vi "basic_movement.vi"() -> ()   [LabVIEW 2019]
uses:
  <vilib>/myRIO/Common/Instrument Driver Framework/myRIO v1.0/Encoder/typedefs/Encoder Signal Mode.ctl
  <vilib>/myRIO/Instrument Drivers/Onboard IO/AI/typedefs/AI Reference.ctl
  <vilib>/myRIO/Common/Instrument Driver Framework/Utilities/typedefs/myRIO Generic Hardware Reference.ctl
  <vilib>/myRIO/Common/Instrument Driver Framework/Utilities/typedefs/Hardware Version Enum.ctl
  <vilib>/myRIO/Common/Instrument Driver Framework/Utilities/typedefs/myRIO v1.0 Reference.ctl
  <vilib>/myRIO/Common/Instrument Driver Framework/Utilities/typedefs/Generic FPGA Reference.ctl
  <vilib>/myRIO/Common/Instrument Driver Framework/myRIO v1.0/AI/typedefs/AI Channels List.ctl
  <vilib>/myRIO/Common/Instrument Driver Framework/myRIO v1.0/AI/typedefs/AI Channels Enum.ctl
  <vilib>/myRIO/Common/Instrument Driver Framework/Utilities/typedefs/Analog Scaling Constants List.ctl
  <vilib>/myRIO/Common/Instrument Driver Framework/Utilities/typedefs/Analog Scaling Constants.ctl
  <vilib>/userDefined/High Color/nirio_resource_hc.ctl
  <vilib>/myRIO/Instrument Drivers/Onboard IO/AO/typedefs/AO Reference.ctl
  <vilib>/myRIO/Common/Instrument Driver Framework/myRIO v1.0/AO/typedefs/AO Channels List.ctl
  <vilib>/myRIO/Common/Instrument Driver Framework/myRIO v1.0/AO/typedefs/AO Channels Enum.ctl
  Shared VIs/TypeDef_TDMS_States.ctl
  <vilib>/Platform/TimedLoop/XDataNode/timing_clust.ctl
  <vilib>/Platform/TimedLoop/XDataNode/nitl_modes.ctl
  <vilib>/Platform/TimedLoop/XDataNode/wakeup.ctl
  <vilib>/myRIO/Common/Instrument Driver Framework/myRIO v1.0/AI/vis/myRIO v1.1 Open AI.vi
  <vilib>/myRIO/Common/Instrument Driver Framework/myRIO v1.0/AO/vis/myRIO v1.1 Open AO.vi
  <vilib>/myRIO/Common/Instrument Driver Framework/Utilities/vis/Validate Channels.vi
  <vilib>/myRIO/Common/Instrument Driver Framework/myRIO v1.0/AI/vis/myRIO v1.0 Reserve AI.vi
  <vilib>/myRIO/Common/Instrument Driver Framework/myRIO v1.0/AO/vis/myRIO v1.0 Reserve AO.vi
  <vilib>/myRIO/Common/Instrument Driver Framework/myRIO v1.0/AI/vis/myRIO v1.0 Close AI.vi
  <vilib>/myRIO/Common/Instrument Driver Framework/myRIO v1.0/Encoder/vis/myRIO v1.0 Close Encoder.vi
  <vilib>/myRIO/Common/Instrument Driver Framework/myRIO v1.0/AO/vis/myRIO v1.0 Close AO.vi
  <vilib>/myRIO/Common/Instrument Driver Framework/myRIO v1.0/AI/vis/myRIO v1.0 Build MUX Configuration AI.vi
  <vilib>/myRIO/Common/Instrument Driver Framework/myRIO v1.0/Resource Manager/vis/myRIO v1.0 Reserve Channel List.vi
  <vilib>/myRIO/Common/Instrument Driver Framework/myRIO v1.0/AO/vis/myRIO v1.0 Build MUX Configuration AO.vi
  <vilib>/myRIO/Common/Instrument Driver Framework/myRIO v1.0/AI/vis/myRIO v1.0 Unreserve AI.vi
  <vilib>/myRIO/Common/Instrument Driver Framework/myRIO v1.0/Encoder/vis/myRIO v1.0 Unreserve Encoder.vi
  <vilib>/myRIO/Common/Instrument Driver Framework/myRIO v1.0/AO/vis/myRIO v1.0 Unreserve AO.vi
  <vilib>/myRIO/Common/Instrument Driver Framework/myRIO v1.0/Resource Manager/vis/myRIO v1.0 Reserve Channel.vi
  <vilib>/myRIO/Common/Instrument Driver Framework/myRIO v1.0/Resource Manager/vis/myRIO v1.0 Unreserve Channel.vi
  <vilib>/myRIO/Common/Instrument Driver Framework/myRIO v1.0/Resource Manager/vis/myRIO v1.0 Unreserve Channel List.vi
  <vilib>/myRIO/Common/Instrument Driver Framework/myRIO v1.0/Encoder/vis/myRIO v1.0 Build MUX Configuration Encoder.vi
  <vilib>/myRIO/Common/Instrument Driver Framework/myRIO v1.0/Resource Manager/vis/myRIO v1.0 Build Mutex Name.vi
  <vilib>/myRIO/Common/Instrument Driver Framework/myRIO v1.0/Resource Manager/vis/myRIO v1.0 Create Configuration List.vi
  <vilib>/Utility/VariantDataType/GetNumericInfo.vi
  <vilib>/Utility/error.llb/Error Cluster From Error Code.vi
  <vilib>/myRIO/Common/Instrument Driver Framework/myRIO v1.0/myRIO v1.1 Open.vi
  <vilib>/myRIO/Common/Instrument Driver Framework/myRIO v1.0/AO/vis/myRIO v1.0 Get Scaling Constants AO.vi
  <vilib>/myRIO/Common/Instrument Driver Framework/Utilities/vis/IO Manager.vi
  <vilib>/myRIO/Common/Instrument Driver Framework/Utilities/vis/Configuration Manager.vi
  <vilib>/myRIO/Common/Instrument Driver Framework/myRIO v1.0/myRIO v1.0 Close.vi
  <vilib>/myRIO/Common/Instrument Driver Framework/myRIO v1.0/AO/vis/myRIO v1.0 Write AO.vi
  <vilib>/myRIO/Common/Instrument Driver Framework/myRIO v1.0/AI/vis/myRIO v1.0 Get Scaling Constants AI.vi
  <vilib>/myRIO/Common/Instrument Driver Framework/myRIO v1.0/AI/vis/myRIO v1.0 Read AI.vi
  <vilib>/myRIO/Common/Instrument Driver Framework/myRIO v1.0/Encoder/vis/myRIO v1.0 Read Encoder.vi
  <vilib>/myRIO/Common/Instrument Driver Framework/myRIO v1.0/Encoder/vis/myRIO v1.0 Enable Encoder.vi
  <vilib>/myRIO/Common/Instrument Driver Framework/myRIO v1.0/Encoder/vis/myRIO v1.0 Shutdown Encoder.vi
  <vilib>/myRIO/Common/Instrument Driver Framework/myRIO v1.0/Resource Manager/vis/myRIO v1.0 Configure IO.vi
  <vilib>/myRIO/Instrument Drivers/Onboard IO/AO/vis/myRIO AO Open.xnode
  <vilib>/myRIO/Instrument Drivers/Onboard IO/AI/vis/myRIO AI Open.xnode
  <vilib>/Platform/TimedLoop/XDataNode/XDataNode.xnode
  <vilib>/myRIO/Instrument Drivers/Onboard IO/Encoder/Encoder.lvlib
  <vilib>/myRIO/Instrument Drivers/Onboard IO/AO/AO.lvlib
  <vilib>/Platform/TimedLoop/XDataNode/XDNodeRunTimeDep.lvlib
  <vilib>/myRIO/Instrument Drivers/Onboard IO/AI/AI.lvlib
panel:
  in  "Save data?":bool
  in  "Stop Saving Data":bool
  in  "Filename Data Save":string
  in  "START":bool
  in  "Motor Input Voltage [V]":dbl
  out "Current (A)":dbl
  out "Loop Number (dt = 1 ms)":dbl
  in  "STOP":bool
  out "Elapsed Time (ms)":dbl
  out "Initial Time (ms)":dbl
  out "Encoder Position (deg)":dbl
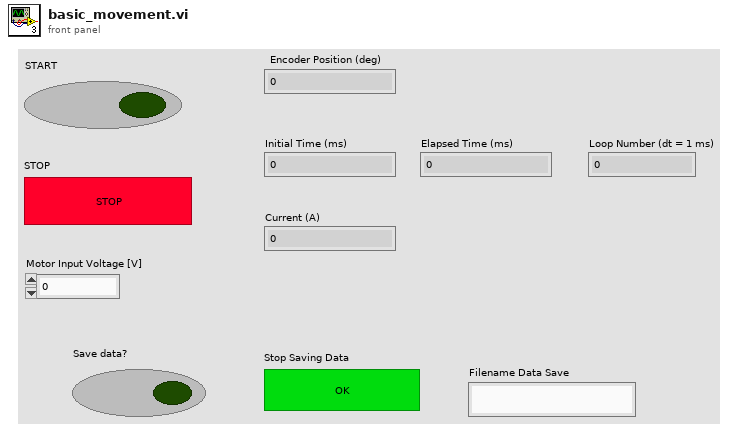
[diagram p1: front panel]
types:
  T1 = typedef "nirio_resource_hc.ctl" = tag
  T2 = typedef "Hardware Version Enum.ctl" = enum16{"Unknown", "myRIO-1900", "myRIO-1950", "roboRIO", "NI ELVIS RIO CM", "ELVIS III"}
  T3 = typedef "TypeDef_TDMS_States.ctl" = enum16{"WaitingForCreate", "Create", "Buffering", "Flushing", "Write", "Close"}
  T4 = enum16{"open", "open or create", "create or replace", "create", "open (read-only)"}
  T5 = typedef "XDNodeRunTimeDep.lvlib/timing_clust.ctl" = cluster{"Expected End [f-1]":u64, "Actual End [f-1]":u64, "Finished Late? [f-1]":bool, "Expected End [i-1]":u64, "Actual End [i-1]":u64, "Finished Late? [i-1]":bool, "Expected Start [i]":u64, "Actual Start [i]":u64, "Expected Start [f]":u64, "Actual Start [f]":u64, "Source Name":string, "Structure Name":string, "Period":i64, "Deadline":i64, "Offset":i64, "Start":i64, "Priority":i32, "Timeout":i32, "Mode":T6, "Wakeup Reason":T7, "Error":errorcluster, "Source Type":string, "Secondary Source Type":string, "Global End Time":u64, "Global Start Time":u64, "Frame Duration":u64, "Iteration Duration":u64, "Assigned CPU":i32, "I/O Scan Engine Mode":u32}
  T6 = typedef "XDNodeRunTimeDep.lvlib/nitl_modes.ctl" = enum32{"No Change", "Process missed periods, maintain original phase", "Discard missed periods, maintain original phase", "Process missed periods, ignore original phase", "Discard missed periods, ignore original phase"}
  T7 = typedef "XDNodeRunTimeDep.lvlib/wakeup.ctl" = enum32{"Normal", "Aborted", "Asynchronous wakeup", "Timing source error", "Timed loop error", "Timeout"}
  T8 = typedef "Encoder Signal Mode.ctl" = enum16{"Quadrature phase signal", "Step and direction signal"}
  T9 = typedef "AO.lvlib/AO Reference.ctl" = cluster{"myRIO Reference":T10, "AO Channel List":T13, "AO Scaling Constant List":T15}
  T10 = typedef "myRIO Generic Hardware Reference.ctl" = cluster{"myRIO Model":T2, "myRIO Hardware Reference":T11}
  T11 = typedef "myRIO v1.0 Reference.ctl" = cluster{"Generic FPGA Reference":T12, "Allow multiple opens":bool}
  T12 = typedef "Generic FPGA Reference.ctl" = refnum<k20>
  T13 = typedef "AO Channels List.ctl" = T14[]
  T14 = typedef "AO Channels Enum.ctl" = enum16{"Not Connected", "AudioOut/Left", "AudioOut/Right", "C/AO0", "C/AO1", "A/AO0", "A/AO1", "B/AO0", "B/AO1"}
  T15 = typedef "Analog Scaling Constants List.ctl" = T16[]
  T16 = typedef "Analog Scaling Constants.ctl" = cluster{"LSB Weight (Volts)":dbl, "Offset (Volts)":dbl, "Signed?":bool}
  T17 = typedef "AI.lvlib/AI Reference.ctl" = cluster{"myRIO Reference":T10, "AI Channels List":T18, "AI Scaling Constants List":T15}
  T18 = typedef "AI Channels List.ctl" = T19[]
  T19 = typedef "AI Channels Enum.ctl" = enum16{"Not Connected", "AudioIn/Left", "AudioIn/Right", "C/AI0", "C/AI1", "A/AI0", "A/AI1", "A/AI2", "A/AI3", "A/AI4", "A/AI5", "A/AI6", "A/AI7", "B/AI0", "B/AI1", "B/AI2", "B/AI3", "B/AI4", "B/AI5", "B/AI6", "B/AI7", "AI/AI0", "AI/AI1", "AI/AI2", "AI/AI3", "A/AI0 (DIFF)", "A/AI1 (DIFF)", "A/AI2 (DIFF)", "A/AI3 (DIFF)", "B/AI0 (DIFF)", "B/AI1 (DIFF)", "B/AI2 (DIFF)", "B/AI3 (DIFF)"}
  T20 = typedef "Encoder.lvlib/Encoder Reference.ctl" = cluster{"myRIO Reference":T10, "Encoder Channels Enum":T21}
  T21 = typedef "Encoder Channels Enum.ctl" = enum16{"Not Connected", "C/ENC0", "C/ENC1", "A/ENC", "A/ENC0", "A/ENC1", "A/ENC2", "A/ENC3", "A/ENC4", "A/ENC5", "A/ENC6", "A/ENC7", "A/ENC8", "A/ENC9", "B/ENC", "B/ENC0", "B/ENC1", "B/ENC2", "B/ENC3", "B/ENC4", "B/ENC5", "B/ENC6", "B/ENC7", "B/ENC8", "B/ENC9", "DIO/ENC0", "DIO/ENC1", "DIO/ENC2", "DIO/ENC3", "DIO/ENC4"}
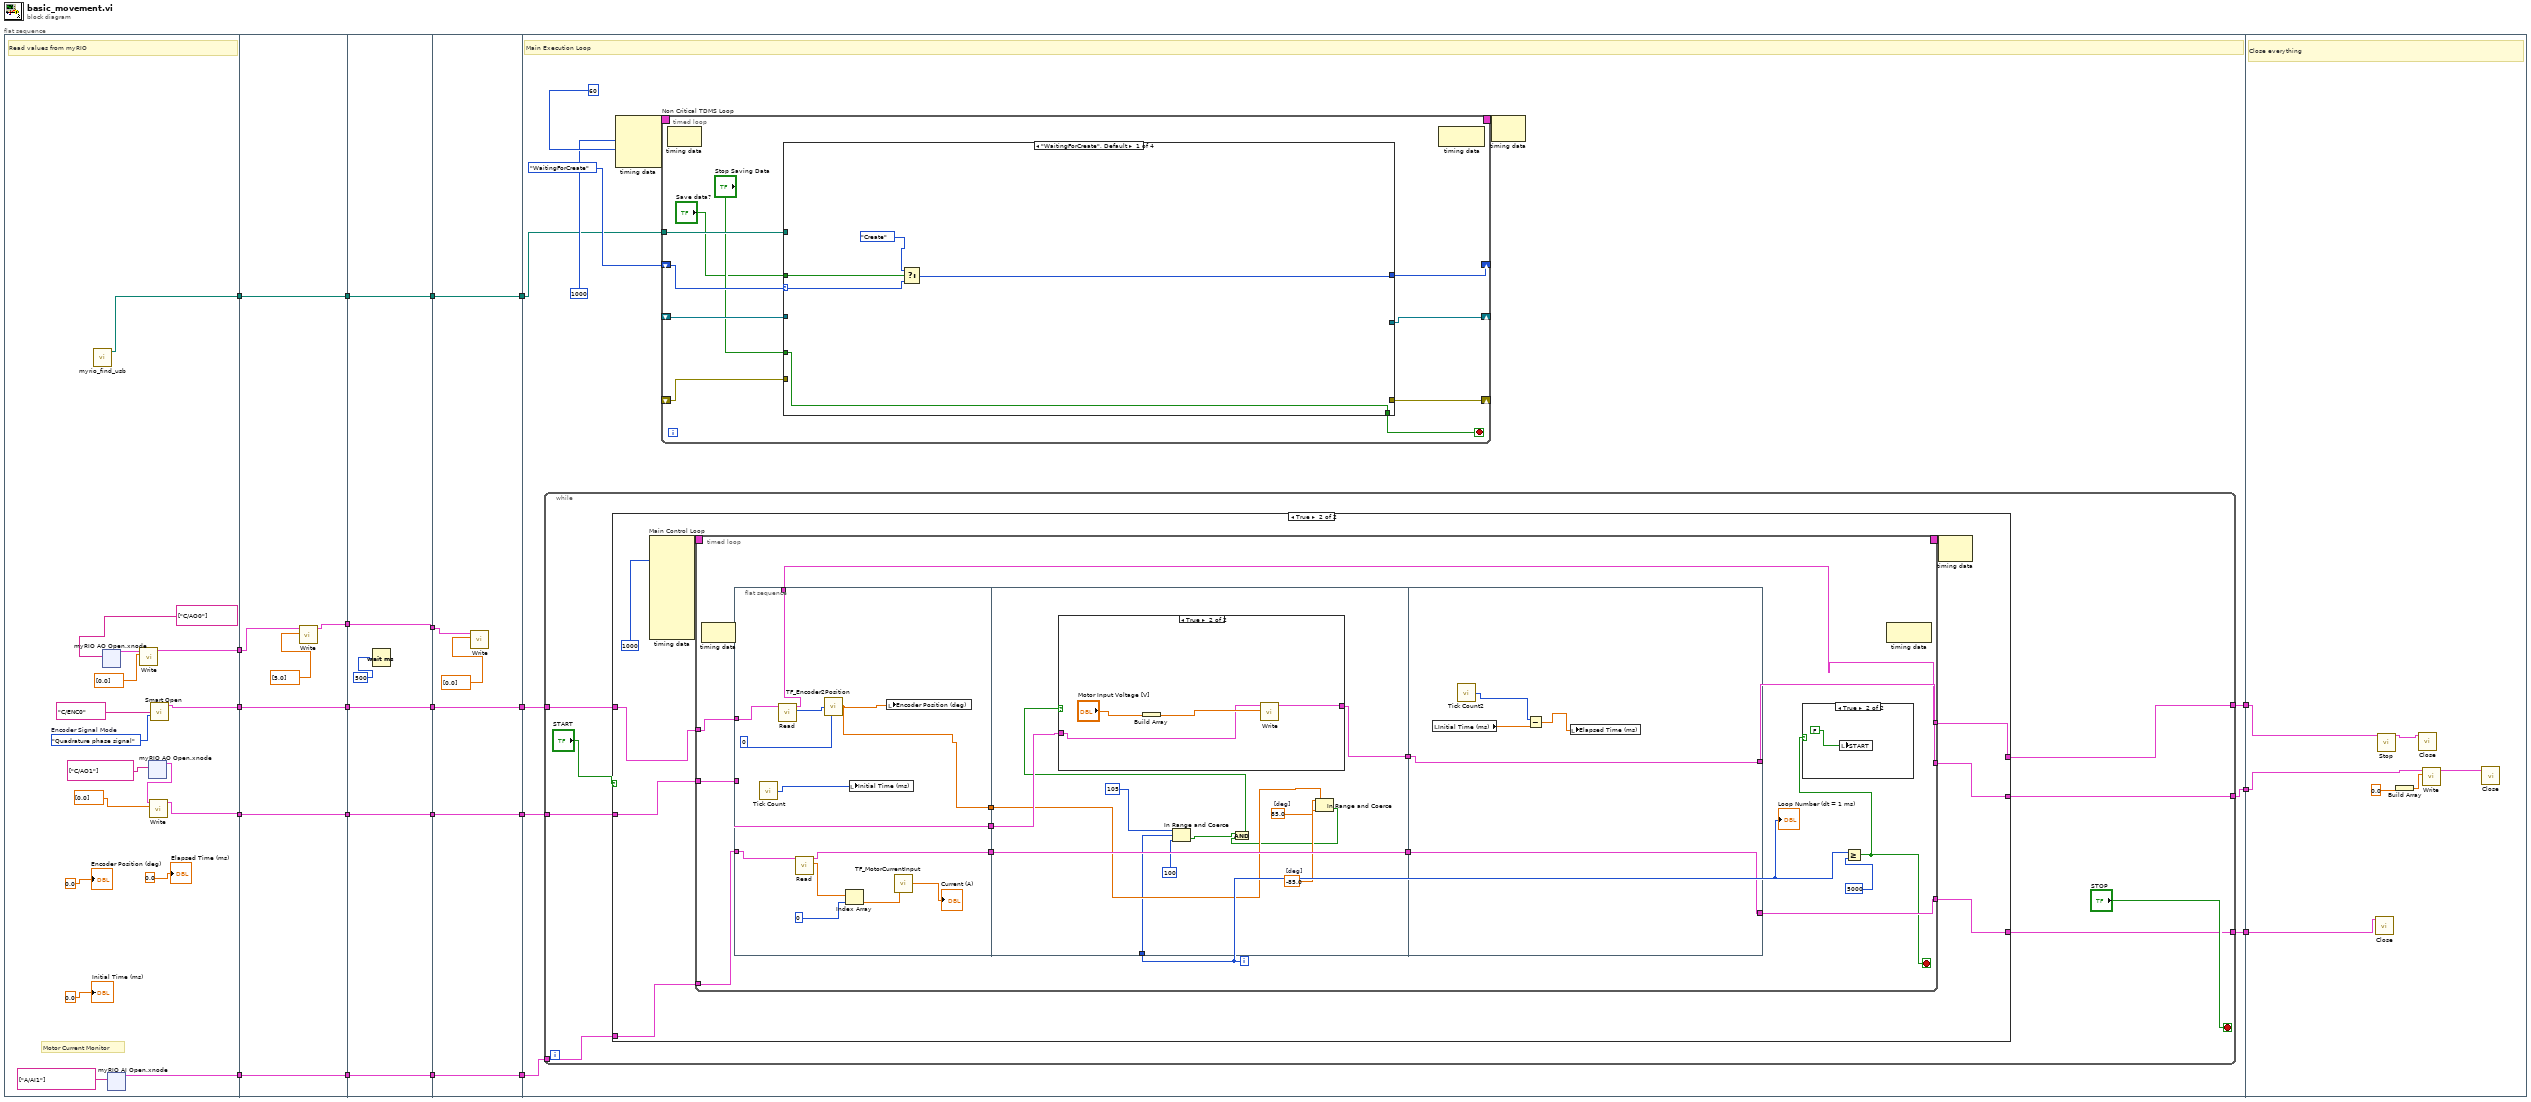
[diagram p0: block diagram]
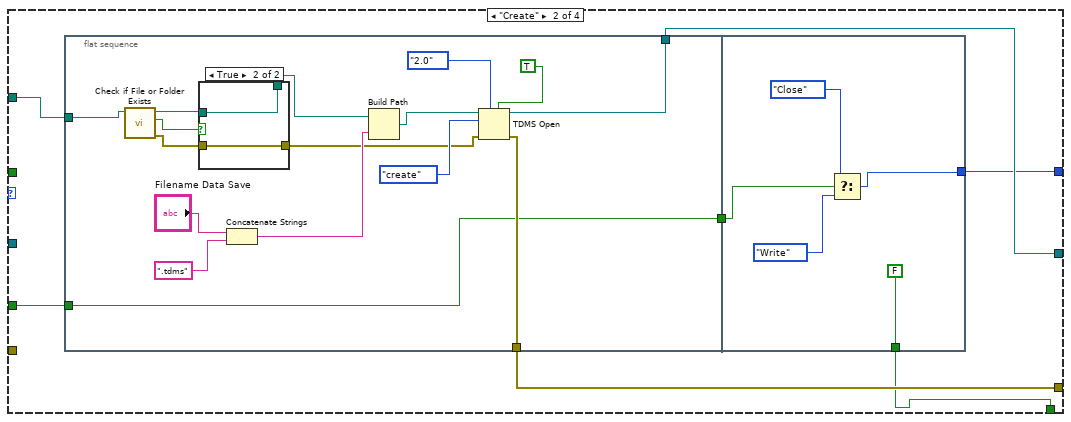
[diagram p2: hidden frame]
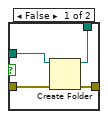
[diagram p3: hidden frame]
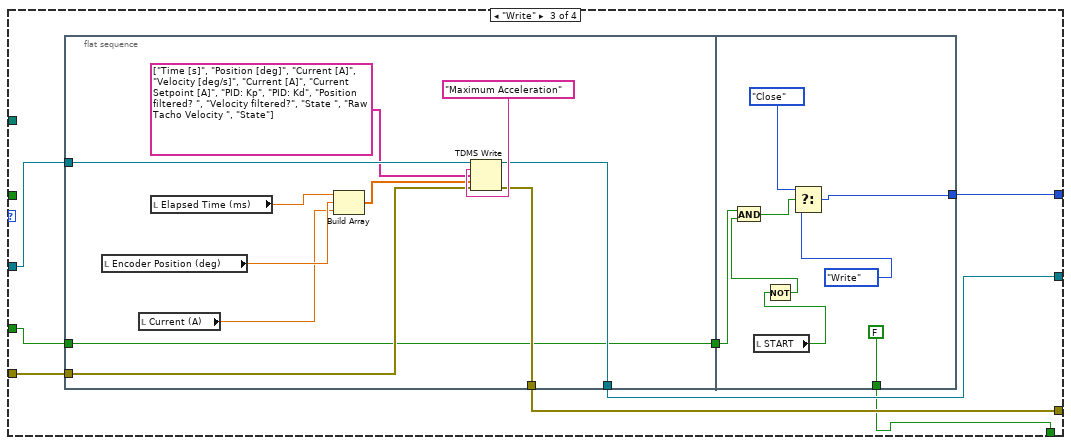
[diagram p4: hidden frame]
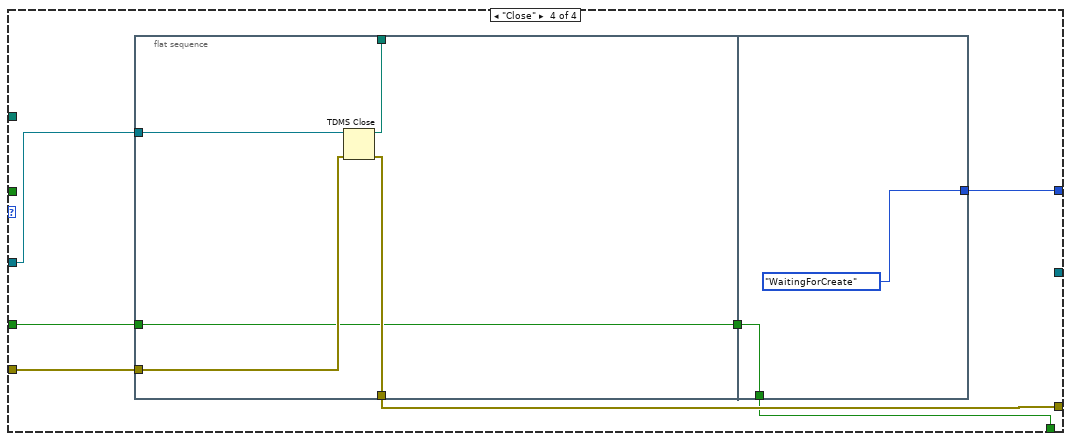
[diagram p5: hidden frame]
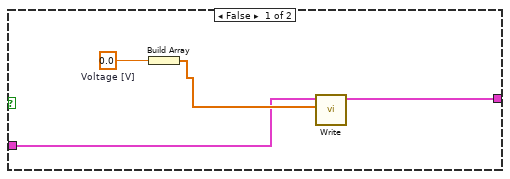
[diagram p8: hidden frame]
diagram:
  n1 = flat-sequence {
    tunnel: [w31] -> w15
    tunnel: [w30] -> w13
    tunnel: [w26] -> w11
    tunnel: [w24] -> w6
    tunnel: [w23] -> w1
    tunnel: w15 -> [w100]
    tunnel: [w100] -> w14
    tunnel: w13 -> [w99]
    tunnel: [w99] -> w12
    tunnel: w11 -> [w97]
    tunnel: [w96] -> w10
    tunnel: [w95] -> w7
    tunnel: w6 -> [w95]
    tunnel: [w94] -> w2
    tunnel: w1 -> [w94]
    tunnel: w14 -> [w106]
    tunnel: [w106] -> w20
    tunnel: w12 -> [w105]
    tunnel: [w105] -> w18
    tunnel: [w103] -> w16
    tunnel: w10 -> [w103]
    tunnel: [w102] -> w8
    tunnel: w7 -> [w102]
    tunnel: [w101] -> w3
    tunnel: w2 -> [w101]
    tunnel: w20 -> [w112]
    tunnel: [w112] -> w19
    tunnel: w18 -> [w111]
    tunnel: [w111] -> w17
    tunnel: w16 -> [w110]
    tunnel: [w108] -> w9
    tunnel: w8 -> [w108]
    tunnel: [w107] -> w4
    tunnel: w3 -> [w107]
    tunnel: w19 -> [w123]
    tunnel: w17 -> [w124]
    tunnel: [w121] -> w22
    tunnel: [w122] -> w21
    tunnel: w9 -> [w120]
    tunnel: [w119] -> w5
    tunnel: w4 -> [w113]
    tunnel: w22 -> [w303]
    tunnel: w21 -> [w302]
    tunnel: w5 -> [w301]
    frame #0 {
      w38 = Encoder_Signal_Mode."Quadrature phase signal"  # Encoder Signal Mode
      # "Motor Current Monitor"
      # "Read values from myRIO"
      n2 = call "myrio_find_usb.vi"() -> ("Largest USB Partition Path"=w23:path)  [unwired: 9 in, 2 out]
      n3 = xnode "myRIO AO Open.xnode"("Channel Names"=tag[] ["C/AO0"]) -> ("AO Ref Out"=w29:T9)  [unwired: 2 in, 1 out]
      n4 = xnode "myRIO AI Open.xnode"("Channel Names"=tag[] ["A/AI1"]) -> ("AI Ref Out"=w24:T17)  [unwired: 2 in, 1 out]
      n5 = call <vilib>:"Write.vi"("Values"=dbl[] [0.0], "AO Ref In"=w29) -> ("AO Ref Out"=w26:T9)  [unwired: 7 in, 1 out]
      n6 = xnode "myRIO AO Open.xnode"("Channel Names"=tag[] ["C/AO1"]) -> ("AO Ref Out"=w36:T9)  [unwired: 2 in, 1 out]
      n7 = call <vilib>:"Write.vi"("Values"=dbl[] [0.0], "AO Ref In"=w36) -> ("AO Ref Out"=w30:T9)  [unwired: 7 in, 1 out]
      n8 = call <vilib>:"Smart Open.vi"("Encoder Signal Mode"=w38, "Channel Name"=tag "C/ENC0") -> ("Encoder Ref Out"=w31:T20)  [unwired: 8 in, 1 out]
      "Encoder Position (deg)" <- 0.0
      "Initial Time (ms)" <- 0.0
      "Elapsed Time (ms)" <- 0.0
    }
    frame #1 {
      n9 = call <vilib>:"Write.vi"("Values"=dbl[] [5.0], "AO Ref In"=w97) -> ("AO Ref Out"=w96:T9)  [unwired: 7 in, 1 out]
    }
    frame #2 {
      n10 = Wait (ms)(milliseconds to wait=500) -> ()  [unwired: 1 out]
    }
    frame #3 {
      n11 = call <vilib>:"Write.vi"("Values"=dbl[] [0.0], "AO Ref In"=w110) -> ()  [unwired: 7 in, 2 out]
    }
    frame #4 {
      # "Main Execution Loop"
      n12 = while {
        tunnel: w124 -> [w229]
        tunnel: w123 -> [w228]
        tunnel: [w225] -> w122
        tunnel: [w226] -> w121
        tunnel: w120 -> [w224]
        tunnel: [w223] -> w119
        stop <- "STOP" stop-if-true
        n13 = case shown="True" "START" {
          tunnel: w229 -> [w231 w238]
          tunnel: w228 -> [w232 w237]
          tunnel: [w231 w236] -> w226
          tunnel: [w232 w235] -> w225
          tunnel: w224 -> [w230 w234]
          tunnel: [w230 w233] -> w223
          frame False {
          }
          frame True {
            n14 = node-c288(1000) -> (w241:T5)  [unwired: 9 in]
            n15 = timed-loop "Main Control Loop" {
              timing: w241 -> [_]
              timing-out: [_] -> w240
              tunnel: w237 -> [w255]
              tunnel: w238 -> [w254]
              tunnel: [w251] -> w236
              tunnel: [w250] -> w235
              tunnel: w234 -> [w249]
              tunnel: [w246] -> w233
              i -> [w244]
              stop <- w242 stop-if-true
              n16 = node-c288() -> ()  [unwired: 1 in, 1 out]
              n17 = flat-sequence {
                tunnel: w255 -> [w267]
                tunnel: w254 -> [w266]
                tunnel: [w266] -> w253
                tunnel: [w265] -> w250
                tunnel: w249 -> [w263]
                tunnel: [w258] -> w247
                tunnel: [w257] -> w245
                tunnel: w244 -> [w271]
                tunnel: w253 -> [w281]
                tunnel: [w280] -> w252
                tunnel: [w279] -> w248
                tunnel: w247 -> [w279]
                tunnel: w245 -> [w276]
                tunnel: w252 -> [w292]
                tunnel: [w292] -> w251
                tunnel: [w290] -> w246
                tunnel: w248 -> [w290]
                frame #0 {
                  n18 = call "Tick Count"() -> ("Tick Count(mSec)"=w264:u32)
                  n19 = call <vilib>:"Read.vi"("Encoder Ref In"=w267) -> ("Counter Value"=w269:i32, "Encoder Ref Out"=w265:T20)  [unwired: 6 in, 3 out]
                  n20 = call <vilib>:"Read.vi"("AI Ref In"=w263) -> ("Values"=w262:dbl[], "AI Ref Out"=w258:T17)  [unwired: 8 in, 1 out]
                  n21 = call "TF_Encoder2Position.vi"("Counter Value"=w269, "Offset"=0) -> ("Position [deg]"=w257:dbl)  [unwired: 3 in]
                  n22 = Index Array(array=w262, index=0) -> (element=w260:dbl)
                  n23 = local write "Initial Time (ms)"(w264) -> ()
                  n24 = local write "Encoder Position (deg)"(w257) -> ()
                  n25 = call "TF_MotorCurrentInput.vi"("Motor Current Monitor Value [V]"=w260) -> ("Current [A]"=→"Current (A)":dbl)
                }
                frame #1 {
                  w277 = 85.0  # [deg]
                  w278 = -85.0  # [deg]
                  n26 = In Range and Coerce(upper limit=105, x=w271, lower limit=100) -> (In Range?=w270:bool)  [unwired: 1 out]
                  n27 = In Range and Coerce(upper limit=w277, x=w276, lower limit=w278) -> (In Range?=w274:bool)  [unwired: 1 out]
                  n28 = And(x=w270, y=w274) -> (x .and. y?=w275:bool)
                  n29 = case shown="True" w275 {
                    tunnel: w281 -> [w283 w288]
                    tunnel: [w282 w287] -> w280
                    frame False {
                      w284 = 0.0  # Voltage [V]
                      n30 = Build Array(w284) -> (w285:dbl[])
                      n31 = call <vilib>:"Write.vi"("Values"=w285, "AO Ref In"=w283) -> ("AO Ref Out"=w282:T9)  [unwired: 7 in, 1 out]
                    }
                    frame True {
                      n32 = Build Array("Motor Input Voltage [V]") -> (w289:dbl[])
                      n33 = call <vilib>:"Write.vi"("Values"=w289, "AO Ref In"=w288) -> ("AO Ref Out"=w287:T9)  [unwired: 7 in, 1 out]
                    }
                  }
                }
                frame #2 {
                  n34 = local read "Initial Time (ms)"() -> (w294:dbl)
                  n35 = call "Tick Count2"() -> ("Tick Count(mSec)"=w291:u32)
                  n36 = Subtract(x=w291, y=w294) -> (x-y=w293:dbl)
                  n37 = local write "Elapsed Time (ms)"(w293) -> ()
                }
              }
              n38 = Greater Or Equal?(x=w244, y=5000) -> (x >= y?=w242:bool)
              n39 = case shown="True" w242 {
                frame False {
                }
                frame True {
                  n40 = local write "START"(FALSE) -> ()
                }
              }
              n41 = node-c288() -> ()  [unwired: 1 in, 1 out]
              "Loop Number (dt = 1 ms)" <- w244
            }
            n42 = node-c288(w240) -> ()  [unwired: 1 out]
          }
        }
      }
      n43 = node-c288(1000, 60) -> (w118:T5)  [unwired: 2 in]
      n44 = timed-loop "Non Critical TDMS Loop" {
        timing: w118 -> [_]
        timing-out: [_] -> w117
        shift-right: [w134] -> _
        shift-left: TypeDef_TDMS_States."WaitingForCreate" ("TDMS States") -> [w133]
        tunnel: w113 -> [w131]
        shift-right: [w130] -> _
        shift-left: _ -> [w127]
        shift-right: [w129] -> _
        shift-left: _ -> [w128]
        stop <- w132 stop-if-true
        n45 = node-c288() -> ()  [unwired: 1 in, 1 out]
        n46 = case shown="\"WaitingForCreate\", Default" w133 {
          selector: w133 -> [w137 _ _ _]
          tunnel: "Save data?" -> [w139 _ _ _]
          tunnel: [w136 w143 w177 w204] -> w134
          tunnel: [w135 w142 w176 w201] -> w132
          tunnel: w131 -> [_ w146 _ _]
          tunnel: [_ w145 w179 w205] -> w130
          tunnel: [_ w144 w178 _] -> w129
          tunnel: w128 -> [_ _ w181 w207]
          tunnel: w127 -> [_ _ w180 w206]
          tunnel: "Stop Saving Data" -> [w135 w140 w174 w202]
          frame "WaitingForCreate", Default {
            n47 = Select(t=TypeDef_TDMS_States."Create" ("TDMS States"), s=w139, f=w137) -> (s? t:f=w136:T3)
          }
          frame "Create" {
            n48 = flat-sequence {
              tunnel: w146 -> [w162]
              tunnel: [w149] -> w145
              tunnel: [w148] -> w144
              tunnel: [w147] -> w141
              tunnel: w140 -> [w147]
              tunnel: [w171] -> w143
              tunnel: [FALSE] -> w142
              tunnel: w141 -> [w169]
              frame #0 {
                n49 = call <vilib>:"Check if File or Folder Exists.vi"("path"=w162) -> ("error out"=w159:errorcluster, "file or folder exists?"=w161:bool, "dup path"=w160:path)  [unwired: 8 in]
                n50 = case shown="True" w161 {
                  tunnel: w160 -> [w166 w167]
                  tunnel: [w165 w168] -> w150
                  tunnel: w159 -> [w164 w168]
                  tunnel: [w163 w167] -> w154
                  frame False {
                    n51 = Create Folder(path (use dialog)=w166, error in=w164) -> (created path=w163:path, error out=w165:errorcluster)  [unwired: 1 in, 1 out]
                  }
                  frame True {
                  }
                }
                n52 = Concatenate Strings("Filename Data Save", ".tdms") -> (w151:string)
                n53 = Build Path(base path=w154, name or relative path=w151) -> (appended path=w158:path)
                n54 = TDMS Open(5:TRUE, 7:enum16{"1.0", "2.0"}."2.0" ("file format version (2.0)"), 8:w150, 10:T4."create" ("operation (0:open)"), 11:w158) -> (0:w149:errorcluster, 3:w148:refnum<k34>)  [unwired: 2 in]
              }
              frame #1 {
                n55 = Select(t=TypeDef_TDMS_States."Close" ("TDMS States"), s=w169, f=TypeDef_TDMS_States."Write" ("TDMS States")) -> (s? t:f=w171:T3)
              }
            }
          }
          frame "Write" {
            n56 = flat-sequence {
              tunnel: w181 -> [w189]
              tunnel: w180 -> [w185]
              tunnel: [w184] -> w179
              tunnel: [w183] -> w178
              tunnel: [w182] -> w175
              tunnel: w174 -> [w182]
              tunnel: [w198] -> w177
              tunnel: [FALSE] -> w176
              tunnel: w175 -> [w196]
              frame #0 {
                n57 = local read "Encoder Position (deg)"() -> (w191:dbl)
                n58 = local read "Current (A)"() -> (w190:dbl)
                n59 = local read "Elapsed Time (ms)"() -> (w192:dbl)
                n60 = Build Array(w192, w191, w190) -> (w186:dbl[])
                n61 = TDMS Write(0:w189, 5:"Maximum Acceleration" ("group name in (Untitled)"), 7:string[] ["Time [s]", "Position [deg]", "Current [A]", "Velocity [deg/s]", "Current [A]", "Current Setpoint [A]", "PID: Kp", "PID: Kd", "Position filtered? ", "Velocity filtered?", "State ", "Raw Tacho Velocity ", "State"], 9:w186, 11:w185) -> (4:w183:refnum<k34>, 15:w184:errorcluster)  [unwired: 1 in, 2 out]
              }
              frame #1 {
                n62 = local read "START"() -> (w195:bool)
                n63 = Not(x=w195) -> (.not. x?=w194:bool)
                n64 = And(x=w196, y=w194) -> (x .and. y?=w193:bool)
                n65 = Select(t=TypeDef_TDMS_States."Close" ("TDMS States"), s=w193, f=TypeDef_TDMS_States."Write" ("TDMS States")) -> (s? t:f=w198:T3)
              }
            }
          }
          frame "Close" {
            n66 = flat-sequence {
              tunnel: w207 -> [w212]
              tunnel: w206 -> [w211]
              tunnel: [w210] -> w205
              tunnel: [w209] -> _
              tunnel: [w208] -> w203
              tunnel: w202 -> [w208]
              tunnel: [TypeDef_TDMS_States."WaitingForCreate" ("TDMS States")] -> w204
              tunnel: w203 -> [w213]
              tunnel: [w213] -> w201
              frame #0 {
                n67 = TDMS Close(8:w211, 11:w212) -> (0:w210:errorcluster, 3:w209:path)
              }
              frame #1 {
              }
            }
          }
        }
        n68 = node-c288() -> ()  [unwired: 1 in, 1 out]
      }
      n69 = node-c288(w117) -> ()  [unwired: 1 out]
    }
    frame #5 {
      # "Close everything"
      n70 = call <vilib>:"Close.vi"("AI Ref In"=w301) -> ()  [unwired: 10 in, 1 out]
      n71 = call <vilib>:"Stop.vi"("Encoder Ref In"=w302) -> ("Encoder Ref Out"=w307:T20)  [unwired: 9 in, 1 out]
      n72 = Build Array(0.0) -> (w304:dbl[])
      n73 = call <vilib>:"Close.vi"("Encoder Ref In"=w307) -> ()  [unwired: 10 in, 1 out]
      n74 = call <vilib>:"Write.vi"("Values"=w304, "AO Ref In"=w303) -> ("AO Ref Out"=w306:T9)  [unwired: 7 in, 1 out]
      n75 = call <vilib>:"Close.vi"("AO Ref In"=w306) -> ()  [unwired: 10 in, 1 out]
    }
  }
